vi "inverse_kin.vi"(6 "Reset":bool, 7 "Parameters":T1={"Stimulus"={"Type"=enum."Off", "Phase"=0.0, "Amplitude"=[0.0, 0.0, 0.0], "Injection point"=enum."Total pose", "Closed loop"=FALSE, "Offset"=[0.0, 0.0, 0.0], "Tip -> world"=TRUE, "Frequency"=0.0, "Length"=0.0}, "Goal Filter A"={"Speedup max"=0.0, "Speedup thresh"=0.15, "Speedup nonlin"=0.0, "Filters"=[]}, "Mode controls"={"Hold"=FALSE, "Cancellation"=FALSE, "Goal filter"=FALSE, "Trigger"=FALSE}, "Manipulator type"=enum."Current piezo", "Manipulator calibration"={"Tool offsets"=[[-1.094526e+33, -1.7368205, -2.1260294e-25]], "Tip light calibration"=[[3.2813332, 0.23462732, 0.17832138, -8265.082], [-0.20249099, 2.693321, -0.28150028, -33565.66], [-0.1458117, 0.68216485, 0.8833545, 26862.188], [-1.1202011e-18, 5.861468e-19, 1.7601345e-18, 1.0]], "Handle light calibration"=[], "Base pivots"=[], "Output pivots"=[[0.0, 0.0, -11360.0]], "Length center"=0.0, "Workspace height"=[], "Workspace diameter"=[0.0, 0.0, 36200.0], "Linearization"=[[0.0, 0.0, 36200.0]], "Stack travel"=400.0, "Saturation pos"=375.0, "Inverse filters"=[]}, "Network"={"Remote Host"="192.168.1.3", "Send Status"=TRUE, "Send Port"=50, "Recv Commands"=FALSE, "Recv Port"=0}, "Goal Filter B"={"Speedup max"=1.0, "Speedup thresh"=2.0, "Speedup nonlin"=0.0, "Filters"=[]}, "Cancellation"={"KP"={"XY"=0.0, "Rxy"=0.0, "Z"=0.0, "Rz"=0.0}, "KI"=2.0, "KD"={"XY"=0.0, "Rxy"=0.0, "Z"=0.0, "Rz"=0.0}, "Max vel"=20.0, "Max acc"=61557.0, "Int error limit"=2.0, "RCM gain"=0.0, "Bypass"=FALSE, "Degraded gain"=0.0}, "Transition time"=3.0, "Estimation"={"Link"={"Measure noise"=[], "Process noise"=[], "Alt process noise"=[], "Alt turnoff cycles"=20, "Innovation limit"=[], "Residue threshold"=0.0, "Enable"=FALSE}, "Handle"={"Measure noise"=[], "Process noise"=[], "State limits"=[], "Innovation limit"=[], "Prediction Lookahead"=0.0, "Enable"=FALSE}}} {"Transition time" format="%_3f"; "Cancellation"."Degraded gain" min=0 max=1 step=0.1 format="%#_3p"; "Cancellation"."RCM gain" min=0 max=1 step=0.1 format="%#_3p"; "Cancellation"."KD"."Rz" min=0 max=1 step=0.1 format="%#_3p"; "Cancellation"."KD"."Rxy" min=0 max=1 step=0.1 format="%#_3p"; "Cancellation"."KD"."Z" min=0 max=1 step=0.1 format="%#_3p"; "Cancellation"."KD"."XY" min=0 max=1 step=0.1 format="%#_3p"; "Cancellation"."KI" min=0 max=1 step=0.01 format="%#_3p"; "Cancellation"."KP"."Rz" min=0 max=1 step=0.1 format="%#_3p"; "Cancellation"."KP"."Rxy" min=0 max=1 step=0.1 format="%#_3p"; "Cancellation"."KP"."Z" min=0 max=1 step=0.1 format="%#_3p"; "Cancellation"."KP"."XY" min=0 max=1 step=0.1 format="%#_3p"; "Cancellation"."Max acc" format="%#_3p"; "Goal Filter B"."Filters"."V limit range" format="%_3p"; "Goal Filter B"."Filters"."V limit" format="%_3p"; "Goal Filter B"."Filters"."Upper Q" format="%_3f"; "Goal Filter B"."Filters"."Upper Fc" format="%_3p"; "Goal Filter B"."Filters"."Lower Q" format="%_3f"; "Goal Filter B"."Filters"."Scale factor" format="%_3f"; "Goal Filter B"."Filters"."Lower Fc" format="%_3p"; "Goal Filter B"."Speedup nonlin" format="%_3p"; "Goal Filter B"."Speedup thresh" format="%_3p"; "Goal Filter B"."Speedup max" format="%_3p"; "Manipulator calibration"."Saturation pos" format="%#.1f"; "Manipulator calibration"."Stack travel" format="%#.1f"; "Manipulator calibration"."Output pivots" format="%#_6f"; "Manipulator calibration"."Base pivots" format="%#_6f"; "Manipulator calibration"."Handle light calibration" format="%#.1f"; "Manipulator calibration"."Tip light calibration" format="%#.1f"; "Goal Filter A"."Filters"."V limit range" format="%_3p"; "Goal Filter A"."Filters"."V limit" format="%_3p"; "Goal Filter A"."Filters"."Upper Q" format="%_3f"; "Goal Filter A"."Filters"."Upper Fc" format="%_3p"; "Goal Filter A"."Filters"."Lower Q" format="%_3f"; "Goal Filter A"."Filters"."Scale factor" format="%_3f"; "Goal Filter A"."Filters"."Lower Fc" format="%_3p"; "Goal Filter A"."Speedup nonlin" format="%_3p"; "Goal Filter A"."Speedup thresh" format="%_3p"; "Goal Filter A"."Speedup max" format="%_3p"; "Stimulus"."Length" min=0.0 max=100.0 step=100.0 format="%#_4p"; "Stimulus"."Frequency" min=0.0 step=100.0 format="%#_4g"; "Stimulus"."Offset" format="%#_3p"; "Stimulus"."Amplitude" format="%#_3p"; "Stimulus"."Phase" min=-180.0 max=360.0 step=100.0 format="%#.2f"}, 8 "Last controller out":sgl[](array[numeric]), 9 "Relative tip motion":sgl[](array[numeric])) -> (0 "Saturation":bool, 1 "Stack motion":sgl[](array[numeric]))   [LabVIEW 2013]
uses:
  <vilib>/Analysis/NI_AALBase.lvlib
  <vilib>/Analysis/baseanly.llb/A x Vector.vi
  testing/injection_point.ctl
  testing/stimulus.ctl
  testing/mode_conrols.ctl
  testing/Micron params.ctl
  asap/labview/testing/probe_calibration.ctl
  host/network_params.ctl
  testing/manipulator_cal.ctl
  filtering/goal_loop_parms.ctl
  decoupled_gain.ctl
  sq_control_params.ctl
  estimation_controls.ctl
panel:
  in  "Saturation mode":bool
  # "Locals:"
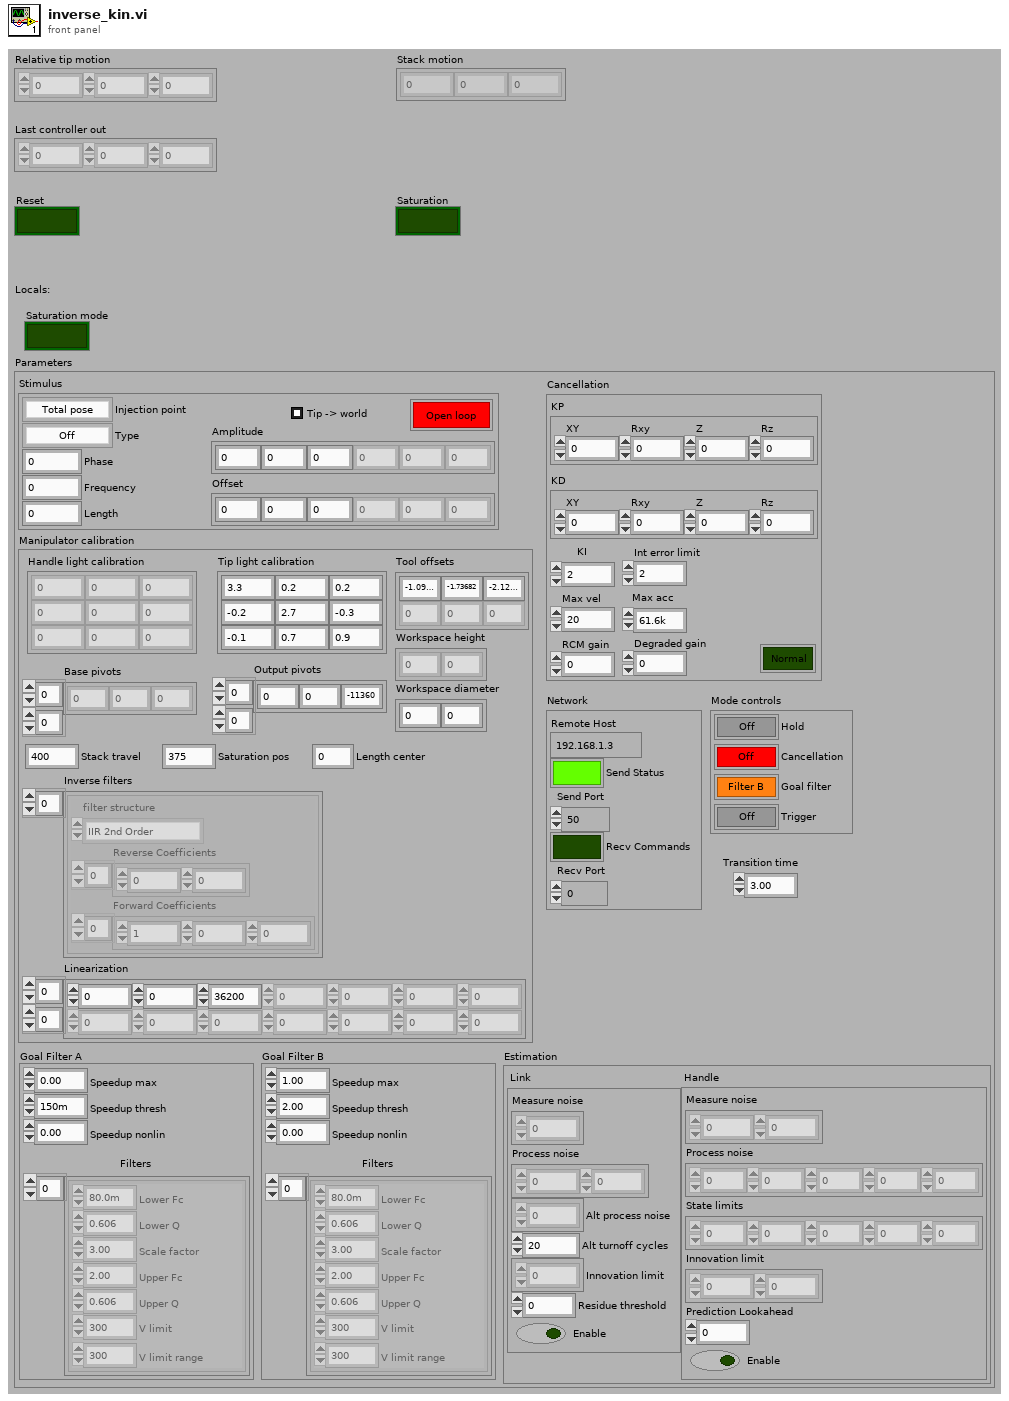
[diagram p1: front panel]
types:
  T1 = typedef "Micron params.ctl" = cluster{"Stimulus":T2, "Goal Filter A":T4, "Mode controls":T5, "Manipulator type":enum16{"Current piezo", "Voltage piezo"}, "Manipulator calibration":T6, "Network":T8, "Goal Filter B":T4, "Cancellation":T9, "Transition time":sgl, "Estimation":T11}
  T2 = typedef "stimulus.ctl" = cluster{"Type":enum16{"Off", "Step", "Sine", "Triangle", "Arbitrary"}, "Phase":dbl, "Amplitude":sgl[], "Injection point":T3, "Closed loop":bool, "Offset":sgl[], "Tip -> world":bool, "Frequency":dbl, "Length":dbl}
  T3 = typedef "injection_point.ctl" = enum16{"Total pose", "V limiter", "Goal ", "Link position", "KF link position", "Inverse kin", "Link goal", "Link error", "Controller", "Output", "Drive", "Light"}
  T4 = typedef "goal_loop_parms.ctl" = cluster{"Speedup max":sgl, "Speedup thresh":sgl, "Speedup nonlin":sgl, "Filters":cluster{"Lower Fc":sgl, "Lower Q":sgl, "Scale factor":sgl, "Upper Fc":sgl, "Upper Q":sgl, "V limit":sgl, "V limit range":sgl}[]}
  T5 = typedef "mode_conrols.ctl" = cluster{"Hold":bool, "Cancellation":bool, "Goal filter":bool, "Trigger":bool}
  T6 = typedef "manipulator_cal.ctl" = cluster{"Tool offsets":sgl[][], "Tip light calibration":T7, "Handle light calibration":T7, "Base pivots":sgl[][], "Output pivots":sgl[][], "Length center":sgl, "Workspace height":sgl[], "Workspace diameter":sgl[], "Linearization":sgl[][], "Stack travel":sgl, "Saturation pos":sgl, "Inverse filters":cluster{"filter structure":enum32{"IIR 2nd Order", "IIR 4th Order"}, "Reverse Coefficients":dbl[], "Forward Coefficients":dbl[]}[]}
  T7 = typedef "probe_calibration.ctl" = sgl[][]
  T8 = typedef "network_params.ctl" = cluster{"Remote Host":string, "Send Status":bool, "Send Port":u16, "Recv Commands":bool, "Recv Port":u16}
  T9 = typedef "sq_control_params.ctl" = cluster{"KP":T10, "KI":sgl, "KD":T10, "Max vel":sgl, "Max acc":sgl, "Int error limit":sgl, "RCM gain":sgl, "Bypass":bool, "Degraded gain":sgl}
  T10 = typedef "decoupled_gain.ctl" = cluster{"XY":sgl, "Rxy":sgl, "Z":sgl, "Rz":sgl}
  T11 = typedef "estimation_controls.ctl" = cluster{"Link":cluster{"Measure noise":dbl[], "Process noise":dbl[], "Alt process noise":dbl[], "Alt turnoff cycles":i32, "Innovation limit":dbl[], "Residue threshold":dbl, "Enable":bool}, "Handle":cluster{"Measure noise":dbl[], "Process noise":dbl[], "State limits":dbl[], "Innovation limit":dbl[], "Prediction Lookahead":sgl, "Enable":bool}}
  T12 = typedef "NI_Matrix.lvlib/RealMatrix.ctl" = dbl[][]
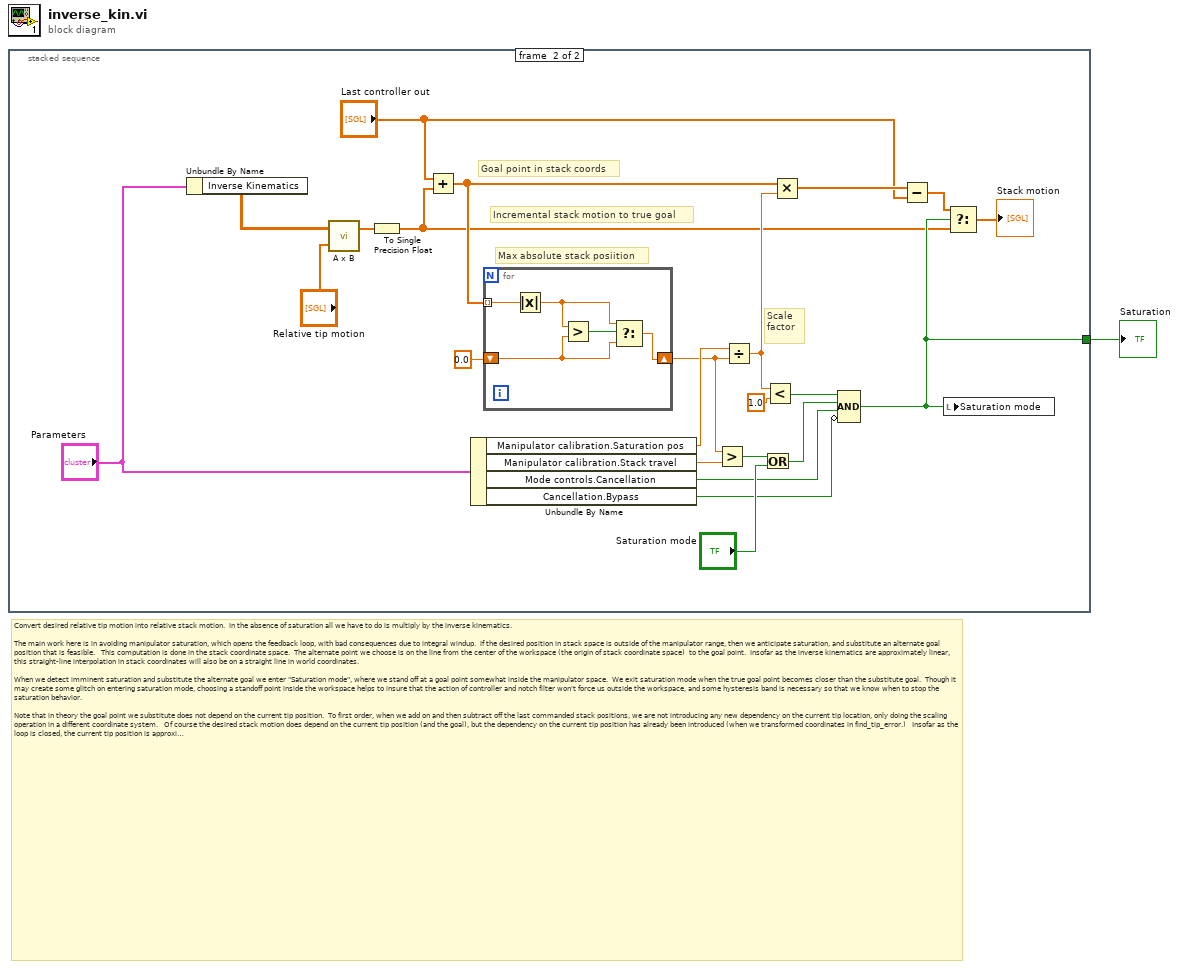
[diagram p0: block diagram]
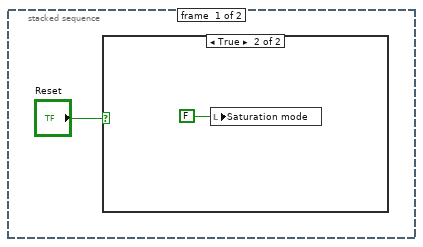
[diagram p2: hidden frame]
diagram:
  # "Convert desired relative tip motion into relative stack motion.  In the absence of saturation all we have to do is multiply by the inverse kinematics.  \n\nThe main work here is in avoiding manipulator saturation, which opens the feedback loop, with bad consequences due to integral windup.  If the desired position in stack space is outside of the manipulator range, then we anticipate saturation, and substitute an alternate goal position that is feasible.   This computation is done in the stack coordinate space.  The alternate point we choose is on the line from the center of the workspace (the origin of stack coordinate space)  to the goal point.  Insofar as the inverse kinematics are approximately linear, this straight-line interpolation in stack coordinates will also be on a straight line in world coordinates.\n\nWhen we detect imminent saturation and substitute the alternate goal we enter \"Saturation mode\", where we stand off at a goal point somewhat inside the manipulator space.  We exit saturation mode when the true goal point becomes closer than the substitute goal.  Though it may create some glitch on entering saturation mode, choosing a standoff point inside the workspace helps to insure that the action of controller and notch filter won't force us outside the workspace, and some hysteresis band is necessary so that we know when to stop the saturation behavior.\n\nNote that in theory the goal point we substitute does not depend on the current tip position.  To first order, when we add on and then subtract off the last commanded stack positions, we are not introducing any new dependency on the current tip location, only doing the scaling operation in a different coordinate system.   Of course the desired stack motion does depend on the current tip position (and the goal), but the dependency on the current tip position has already been introduced (when we transformed coordinates in find_tip_error.)   Insofar as the loop is closed, the current tip position is approximately the goal position, so the current stack positions are approximately the goal point expressed in stack coordinates. \n\nThe reason for substituting a goal point along the line to the true goal is that this creates a smooth transition when we exit saturation mode.   Our interpolation is definitely along a line toward the center of the workspace, but it may not be exactly in the direction of the goal.  This should be acceptable as long we get smooth transitions in and out of saturation mode.  What is perhaps more important for our purposes is that, regardless of the current error between the commanded stack position and actual position (due to slew limiting, etc.), we are closely following the computation that the PID controller uses, so will always choose a position that is not going to drive the manipulator into saturation."
  n1 = stacked-sequence {
    tunnel: [_ w11] -> w1
    frame #0 {
      n2 = case shown="True" "Reset" {
        frame False {
        }
        frame True {
          n3 = local write "Saturation mode"(FALSE ("Saturation mode")) -> ()
        }
      }
    }
    frame #1 {
      # "Incremental stack motion to true goal"
      # "Scale factor"
      # "Max absolute stack posiition"
      # "Goal point in stack coords"
      n4 = Unbundle By Name("Parameters") -> ("Inverse Kinematics"=w25:T12)
      n5 = call-poly <vilib>:"A x B.vi"("Vector"="Relative tip motion", "A"=w25) -> ("A x Vector"=w23:dbl[])  [unwired: 1 out]
      n6 = To Single Precision Float(number=w23) -> (single precision float=w6:sgl[])
      n7 = Add(x="Last controller out", y=w6) -> (x+y=w21:sgl[])
      n8 = Unbundle By Name("Parameters") -> ("Manipulator calibration.Saturation pos"=w20:sgl, "Manipulator calibration.Stack travel"=w18:sgl, "Mode controls.Cancellation"=w10:bool, "Cancellation.Bypass"=w4:bool)
      n9 = for {
        tunnel: w21 -> [w31] mode=indexing
        shift-right: [w27] -> w8
        shift-left: sgl 0.0 -> [w28]
        n10 = Absolute Value(x=w31) -> (abs(x)=w29:sgl)
        n11 = Greater?(x=w29, y=w28) -> (0:w30:bool)
        n12 = Select(t=w29, s=w30, f=w28) -> (s? t:f=w27:sgl)
      }
      n13 = Greater?(x=w8, y=w18) -> (0:w17:bool)
      n14 = Divide(x=w20, y=w8) -> (x/y=w9:sgl)
      n15 = Or(x=w17, y="Saturation mode") -> (x .or. y?=w14:bool)
      n16 = Less?(x=w9, y=sgl 1.0) -> (x < y?=w15:bool)
      n17 = Multiply(x=w21, y=w9) -> (x*y=w7:sgl[])
      n18 = Compound Arithmetic op=AND(w15, w14, w10, invert w4) -> (w11:bool)
      n19 = Subtract(x=w7, y="Last controller out") -> (x-y=w13:sgl[])
      n20 = local write "Saturation mode"(w11) -> ()
      n21 = Select(t=w13, s=w11, f=w6) -> (s? t:f=→"Stack motion":sgl[])
    }
  }
  "Saturation" <- w1
